vi "I32ToString(cast).vi"(1 "U32":u32 format="DEC:%2d\nHEX:%2x") -> (0 "String":string)   [LabVIEW 2012]
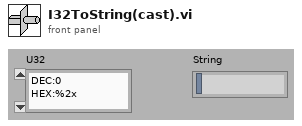
[diagram p1: front panel]
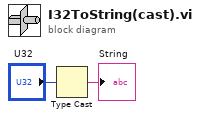
[diagram p0: block diagram]
diagram:
  n1 = Type Cast(x="U32") -> (*(type *) &x=→"String":string)  [unwired: 1 in]
